vi "Init Serial.vi"(7 "Error Checking (Full)":T2=enum."Full", 8 "error in (no error)":errorcluster, 10 "Baud (115200)":u32=115200, 11 "VISA resource name in":refnum<visa-resource-name>) -> (0 "error out":errorcluster, 2 "Identity":T1, 3 "Session":refnum<class "Session.lvclass">)   [LabVIEW 2024, in "CTI.lvlib" / "VisaComms.lvclass"]
uses:
  VisaComms.lvclass
  Session/Session.lvclass
  Error Reporting.ctl
  Identity.ctl
  C:/Users/nkirchne/Documents/~SANDBOX/Electronics Workflow/build/ForPort/CTI/DeviceComms/DeviceComms.lvclass
  CTI.lvlib
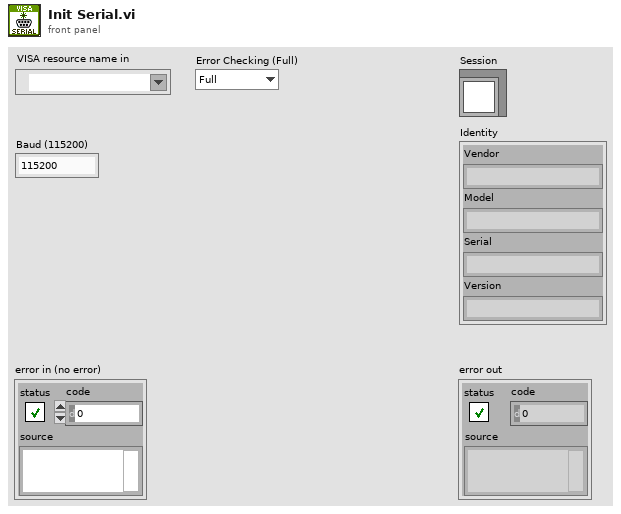
[diagram p1: front panel]
types:
  T1 = typedef "CTI.lvlib/Identity.ctl" = cluster{"Vendor":string, "Model":string, "Serial":string, "Version":string}
  T2 = typedef "CTI.lvlib/Error Reporting.ctl" = enum16{"Minimal", "Moderate", "Full"}
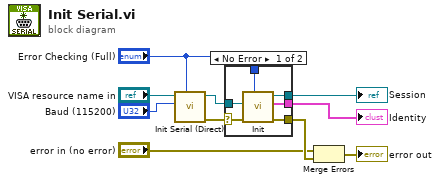
[diagram p0: block diagram]
diagram:
  n1 = call "Init Serial (Direct).vi"("Error Checking (Full)"="Error Checking (Full)", "Baud (115200)"="Baud (115200)", "VISA resource name in"="VISA resource name in") -> ("error out"=w3:errorcluster, "VisaComms out"=w2:refnum<class "VisaComms.lvclass">)  [unwired: 6 in, 1 out]
  n2 = case shown="No Error" w3 {
    selector: w3 -> [w13 w17]
    tunnel: [w16 _] -> w10
    tunnel: [w15 w17] -> w8
    tunnel: w2 -> [w14 _]
    tunnel: "Error Checking (Full)" -> [w12 _]
    tunnel: [w11 _] -> w1
    frame No Error {
      n3 = call "Init.vi"("Error Checking (Full)"=w12, "error in (no error)"=w13, "DeviceComms"=w14) -> ("error out"=w15:errorcluster, "Identity"=w11:T1, "Session out"=w16:refnum<class "Session.lvclass">)  [unwired: 6 in]
    }
    frame Error {
    }
  }
  "Session" <- w10
  "Identity" <- w1
  n4 = Merge Errors("error in (no error)", w8) -> (→"error out":errorcluster)
